vi "Instrument.Oxford1820.Get All.vi"(8 "error in (no error)":errorcluster, 11 "Instrument.Oxford1820 in":refnum<class "Instrument.Oxford1820.lvclass">) -> (0 "error out":errorcluster, 2 "getAll":T1, 3 "Instrument.Oxford1820 out":refnum<class "Instrument.Oxford1820.lvclass">)   [LabVIEW 2019, in "Instrument.Oxford1820.lvclass"]
uses:
  Instrument.Oxford1820.lvclass
  Typedefs/getAll.ctl
  dc0cc8a6-f523-4bfd-92b5-2bd7d48bfea2.vi/ac6a1d9e-6f21-437f-b2a9-999cd16545a3.vi
  dc0cc8a6-f523-4bfd-92b5-2bd7d48bfea2.vi/ac6a1d9e-6f21-437f-b2a9-999cd16545a3.vi/d35817d7-a74a-4219-917f-216192035937.vi
  dc0cc8a6-f523-4bfd-92b5-2bd7d48bfea2.vi/ac6a1d9e-6f21-437f-b2a9-999cd16545a3.vi/fe35985d-5336-47bc-a99d-20060642274b.vi
  dc0cc8a6-f523-4bfd-92b5-2bd7d48bfea2.vi/ac6a1d9e-6f21-437f-b2a9-999cd16545a3.vi/fe35985d-5336-47bc-a99d-20060642274b.vi/de55f414-6d1c-40b3-927a-4e9f6e935836.vi
  dc0cc8a6-f523-4bfd-92b5-2bd7d48bfea2.vi/ac6a1d9e-6f21-437f-b2a9-999cd16545a3.vi/fe35985d-5336-47bc-a99d-20060642274b.vi/282ca4e2-8e31-42cc-b4a8-ed57c7443669.vi
  <userlib>/LevyLab/Levylab Instruments/SMOs/RemoteControl/API/Remote Client.vi
  <vilib>/JDP Science/JSONtext/JSON text to Variant.vi
  <vilib>/JDP Science/JSONtext/LVClass Serializer/JSONtext LVClass Serializer.lvclass
  <userlib>/LevyLab/Levylab Instruments/SMOs/Instrument/Typedefs/Instrument.Commands--Enum.ctl
  <userlib>/LevyLab/Levylab Instruments/SMOs/Instrument/Instrument.lvclass
  2b60fb14-ae40-4096-b3e4-9beee409ef21.vi
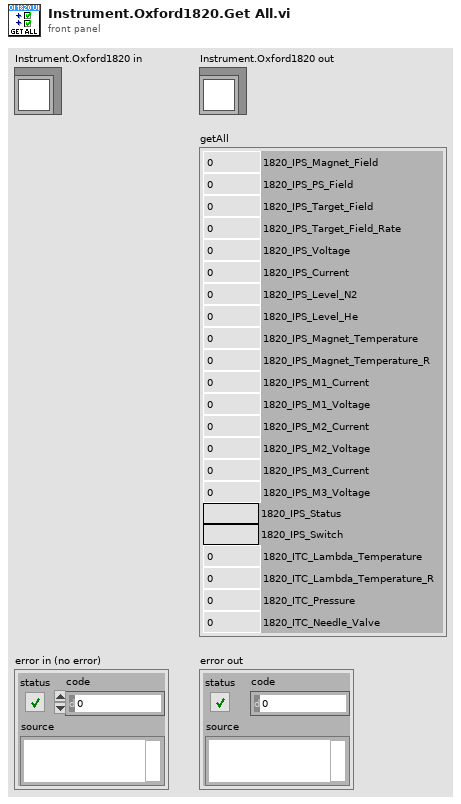
[diagram p1: front panel]
types:
  T1 = typedef "Instrument.Oxford1820.lvclass/getAll.ctl" = cluster{"1820_IPS_Magnet_Field":dbl, "1820_IPS_PS_Field":dbl, "1820_IPS_Target_Field":dbl, "1820_IPS_Target_Field_Rate":dbl, "1820_IPS_Voltage":dbl, "1820_IPS_Current":dbl, "1820_IPS_Level_N2":dbl, "1820_IPS_Level_He":dbl, "1820_IPS_Magnet_Temperature":dbl, "1820_IPS_Magnet_Temperature_R":dbl, "1820_IPS_M1_Current":dbl, "1820_IPS_M1_Voltage":dbl, "1820_IPS_M2_Current":dbl, "1820_IPS_M2_Voltage":dbl, "1820_IPS_M3_Current":dbl, "1820_IPS_M3_Voltage":dbl, "1820_IPS_Status":string, "1820_IPS_Switch":string, "1820_ITC_Lambda_Temperature":dbl, "1820_ITC_Lambda_Temperature_R":dbl, "1820_ITC_Pressure":dbl, "1820_ITC_Needle_Valve":dbl}
  T2 = typedef "Instrument.lvclass/Instrument.Commands--Enum.ctl" = enum16{"HELP", "ACK", "getAll"}
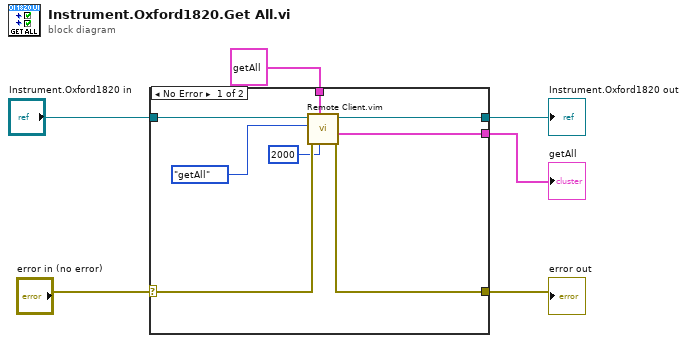
[diagram p0: block diagram]
diagram:
  n1 = case shown="No Error" "error in (no error)" {
    selector: "error in (no error)" -> [w9 w17]
    tunnel: T1 {"1820_IPS_Magnet_Field"=0.0, "1820_IPS_PS_Field"=0.0, "1820_IPS_Target_Field"=0.0, "1820_IPS_Target_Field_Rate"=0.0, "1820_IPS_Voltage"=0.0, "1820_IPS_Current"=0.0, "1820_IPS_Level_N2"=0.0, "1820_IPS_Level_He"=0.0, "1820_IPS_Magnet_Temperature"=0.0, "1820_IPS_Magnet_Temperature_R"=0.0, "1820_IPS_M1_Current"=0.0, "1820_IPS_M1_Voltage"=0.0, "1820_IPS_M2_Current"=0.0, "1820_IPS_M2_Voltage"=0.0, "1820_IPS_M3_Current"=0.0, "1820_IPS_M3_Voltage"=0.0, "1820_IPS_Status"="", "1820_IPS_Switch"="", "1820_ITC_Lambda_Temperature"=0.0, "1820_ITC_Lambda_Temperature_R"=0.0, "1820_ITC_Pressure"=0.0, "1820_ITC_Needle_Valve"=0.0} ("getAll") -> [w12 w15]
    tunnel: [w10 w15] -> w5
    tunnel: [w11 w16] -> w4
    tunnel: "Instrument.Oxford1820 in" -> [w13 w16]
    tunnel: [w8 w17] -> w1
    frame No Error {
      n2 = call "Remote Client.vim"("timeout (ms) [500]"=2000, "Data Out type"=w12, "error in (no error)"=w9, "method"=Instrument.Commands--Enum."getAll" ("Commands"), "Instrument in"=w13) -> ("error out"=w8:errorcluster, "Data out"=w10:T1, "Instrument out"=w11:refnum<class "Instrument.Oxford1820.lvclass">)  [unwired: 3 in, 1 out]
    }
    frame Error {
    }
  }
  "getAll" <- w5
  "Instrument.Oxford1820 out" <- w4
  "error out" <- w1
